vi "Measurement Logic.vi"() -> ()   [LabVIEW 2021, in "audio_adc_acDualChannelMeasurement.lvlib"]
uses:
  audio_adc_acDualChannelMeasurement.lvlib
  Measurement Configuration.ctl
  <vilib>/MeasurementLink/MeasurementLink Measurement Server/Classes/MeasurementContext/MeasurementContext.lvclass
  Measurement Results.ctl
  <vilib>/PDM Acquisition Toolkit/host/Classes/Tasks/PCM Input/Controls/DVR PCM Input Task.ctl
  <vilib>/PDM Acquisition Toolkit/host/Classes/Tasks/PCM Input/PCM Input Task.lvclass
  shared/controls/Sync Commands.ctl
  sub-vis/Protocol Settings Dual Channel.ctl
  <vilib>/DAQmx/create/channels.llb/DAQmx Create Channel (AO-Voltage-Basic).vi
  <vilib>/DAQmx/configure/timing.llb/DAQmx Timing (Sample Clock).vi
  <vilib>/DAQmx/create/channels.llb/DAQmx Create Channel (AO-FuncGen).vi
  <vilib>/PDM Acquisition Toolkit/host/API/Public/Start/Start PCM Input Task.vi
  <vilib>/PDM Acquisition Toolkit/host/API/Public/Read/Read PCM Input Waveform.vi
  <vilib>/PDM Acquisition Toolkit/host/API/Public/Clear/Clear PCM Input Task.vi
  <resource>/objmgr/daqmx.rc
  <vilib>/PDM Acquisition Toolkit/host/API/PDM Acquisition Toolkit.lvlib
panel:
  out "Measurement Results":T1
  out "Measurement Context out":refnum<class "MeasurementContext.lvclass">
  in  "Measurement Context":refnum<class "MeasurementContext.lvclass">
  in  "Measurement Configuration":T2={"Band start"=20.0, "Band stop"=20000.0, "Weighting filter"="", "Amplitude"=1.0, "Frequency"=1000.0, "Full scale range"=2.825, "Analog source resource name"="", "Protocol capture resource name"="", "Data line"=0, "Sample rate"=12288000.0, "Measurement duration"=19200.0, "Channel"="0L", "Frame sync edge for channel 0"=0, "Channel count per frame"=2, "Channel length"=32, "Bit depth"=24, "Channel 0 offset"=1, "Endianness"=0, "Data justification"=0, "Frame length"=64, "Frame sync pulse width"=32, "Bit clock edge sync"=1}
  out "error out":errorcluster
  in  "error in":errorcluster
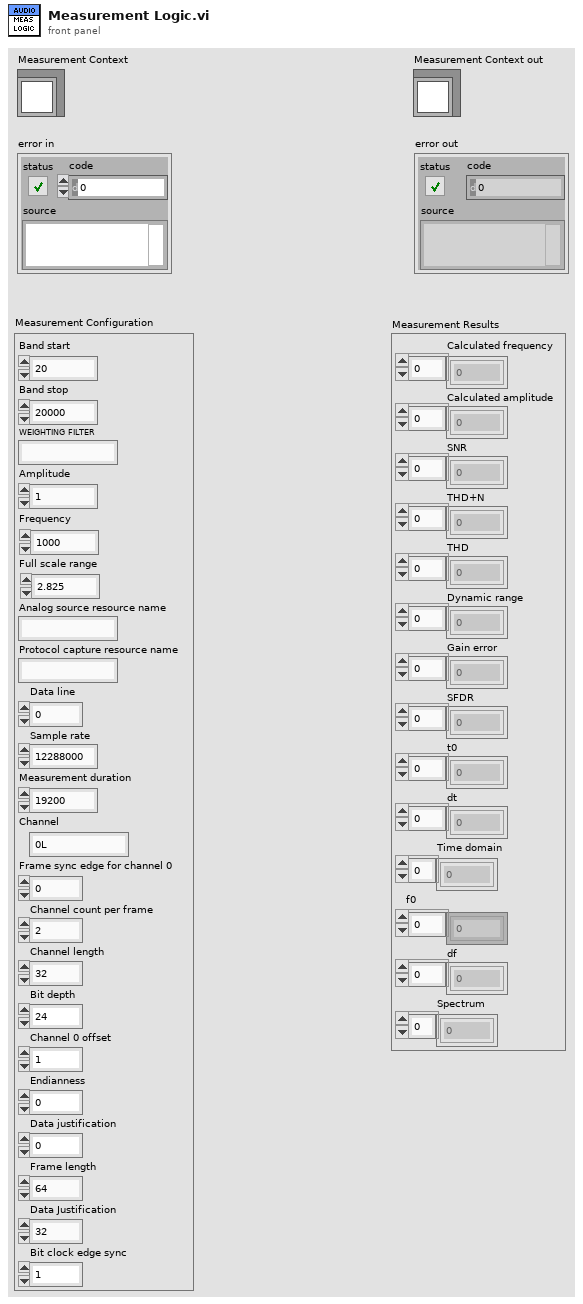
[diagram p1: front panel]
types:
  T1 = typedef "audio_adc_acDualChannelMeasurement.lvlib/Measurement Results.ctl" = cluster{"Calculated frequency":dbl[], "Calculated amplitude":dbl[], "SNR":dbl[], "THD+N":dbl[], "THD":dbl[], "Dynamic range":dbl[], "Gain error":dbl[], "SFDR":dbl[], "t0":dbl[], "dt":dbl[], "Time domain":dbl[], "f0":dbl[], "df":dbl[], "Spectrum":dbl[]}
  T2 = typedef "audio_adc_acDualChannelMeasurement.lvlib/Measurement Configuration.ctl" = cluster{"Band start":dbl, "Band stop":dbl, "Weighting filter":string, "Amplitude":dbl, "Frequency":dbl, "Full scale range":dbl, "Analog source resource name":string, "Protocol capture resource name":string, "Data line":u16, "Sample rate":dbl, "Measurement duration":dbl, "Channel":string, "Frame sync edge for channel 0":u32, "Channel count per frame":u32, "Channel length":u32, "Bit depth":u32, "Channel 0 offset":u32, "Endianness":u32, "Data justification":u32, "Frame length":u32, "Frame sync pulse width":u32, "Bit clock edge sync":u32}
  T3 = typedef "Sync Commands.ctl" = enum16{"NoAction", "GenerationStarted", "AcquisitionCompleted", "GenerationErrored"}
  T4 = typedef "PDM Acquisition Class Library.lvlib/PCM Input Task.lvclass/DVR PCM Input Task.ctl" = refnum<data-value>
  T5 = cluster{"DSG Session":refnum<k21>, "PDM task":T4, "Measurement Results":T1}
  T6 = typedef "audio_adc_acDualChannelMeasurement.lvlib/Protocol Settings Dual Channel.ctl" = cluster{"Protocol capture resource name":string, "Data line":u16, "Channel":string, "Clock rate":u32, "Number of words":i32, "Sensitivity":dbl, "Frame sync edge for channel 0":enum32{"Rising", "Falling"}, "Channel count per frame":u8, "Channel length":u16, "Bit depth":u8, "Channel 0 offset":u16, "Endianness":enum32{"MSB First", "LSB First"}, "Data justification":enum32{"Left Justified", "Right Justified"}, "Frame length":u16, "Frame sync pulse width":u16, "Bit clock edge sync":enum32{"Rising", "Falling"}}
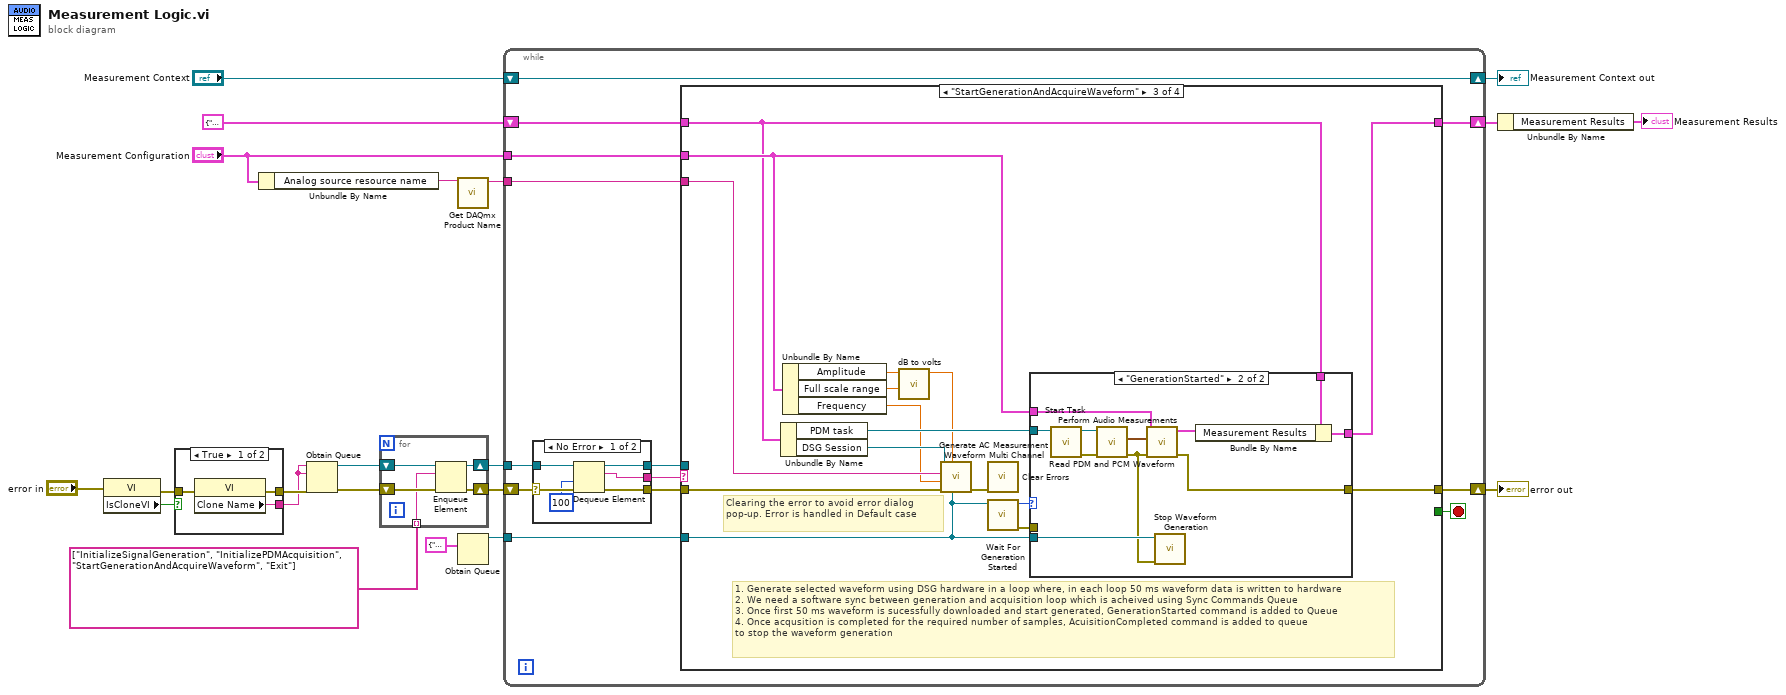
[diagram p0: block diagram]
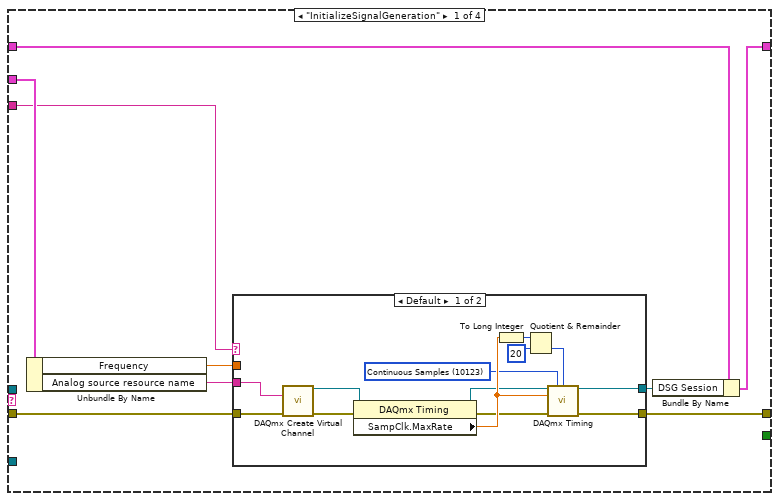
[diagram p2: hidden frame]
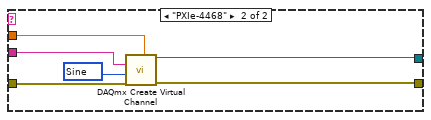
[diagram p3: hidden frame]
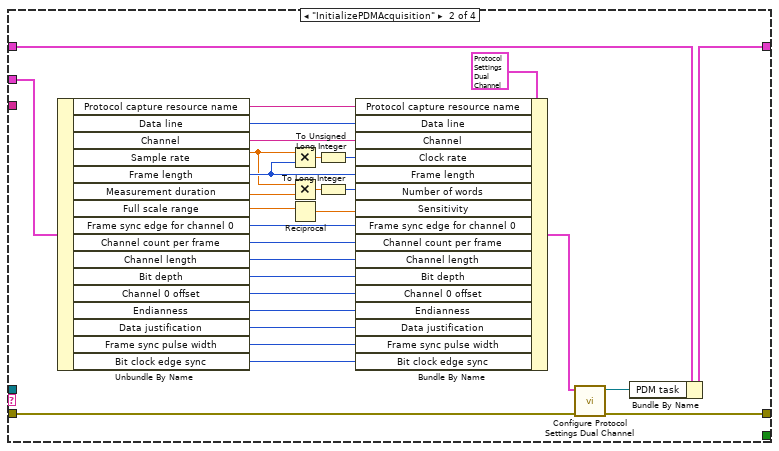
[diagram p4: hidden frame]
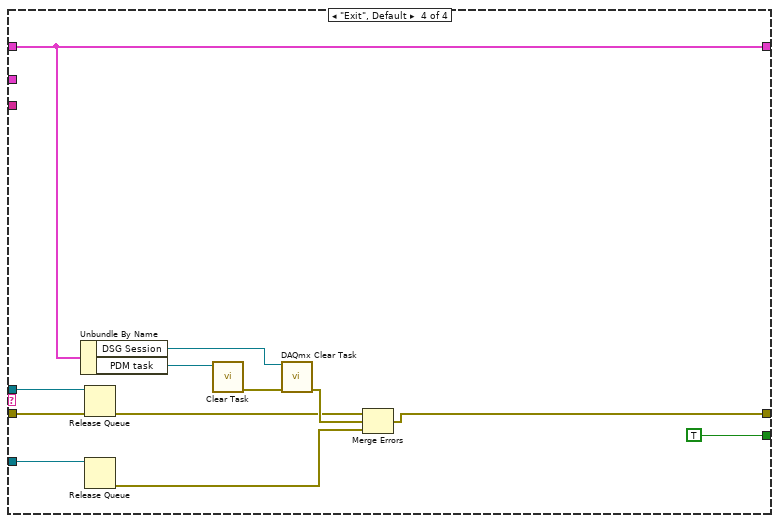
[diagram p6: hidden frame]
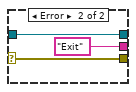
[diagram p7: hidden frame]
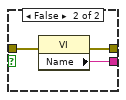
[diagram p8: hidden frame]
diagram:
  n1 = property class="VI"(error in="error in") -> (error out=w19:errorcluster, "IsCloneVI"=w20:bool)  [unwired: 1 in, 1 out]
  n2 = case shown="True" w20 {
    tunnel: [w24 w27] -> w18
    tunnel: [w23 w26] -> w1
    tunnel: w19 -> [w22 w25]
    frame True {
      n3 = property class="VI"(error in=w22) -> (error out=w24:errorcluster, "Clone Name"=w23:string)  [unwired: 1 in, 1 out]
    }
    frame False {
      n4 = property class="VI"(error in=w25) -> (error out=w27:errorcluster, "Name"=w26:string)  [unwired: 1 in, 1 out]
    }
  }
  n5 = Unbundle By Name("Measurement Configuration") -> ("Analog source resource name"=w10:string)
  n6 = Obtain Queue(name (unnamed)=w1, element data type=w1, error in (no error)=w18) -> (queue out=w21:refnum<queue>, error out=w17:errorcluster)  [unwired: 2 in, 1 out]
  n7 = for {
    shift-right: [w30] -> w16
    shift-left: w21 -> [w32]
    shift-right: [w29] -> w15
    shift-left: w17 -> [w31]
    tunnel: string[] ["InitializeSignalGeneration", "InitializePDMAcquisition", "StartGenerationAndAcquireWaveform", "Exit"] ("Step sequence") -> [w28] mode=indexing
    n8 = Enqueue Element(queue=w32, element=w28, error in (no error)=w31) -> (queue out=w30:refnum<queue>, error out=w29:errorcluster)  [unwired: 1 in, 1 out]
  }
  n9 = call "Get DAQmx Product Name.vi"("DAQmx resource name"=w10) -> ("DAQmx product type"=w8:string)  [unwired: 10 in]
  n10 = Obtain Queue(element data type=cluster{"Status":T3, "Error":errorcluster} {"Status"=enum."NoAction", "Error"={"status"=FALSE, "code"=0, "source"=""}}) -> (queue out=w2:refnum<queue>)  [unwired: 4 in, 2 out]
  n11 = while {
    tunnel: w16 -> [w45]
    shift-right: [w42] -> w6
    shift-left: w15 -> [w41]
    shift-right: [w38] -> w11
    shift-left: "Measurement Context" -> [w38]
    tunnel: "Measurement Configuration" -> [w39]
    shift-right: [w36] -> w5
    shift-left: T5 {"DSG Session"="", "PDM task"=refnum, "Measurement Results"={"Calculated frequency"=[], "Calculated amplitude"=[], "SNR"=[], "THD+N"=[], "THD"=[], "Dynamic range"=[], "Gain error"=[], "SFDR"=[], "t0"=[], "dt"=[], "Time domain"=[], "f0"=[], "df"=[], "Spectrum"=[]}} -> [w40]
    tunnel: w8 -> [w35]
    tunnel: w2 -> [w34]
    stop <- w37 stop-if-true
    n12 = case shown="No Error" w41 {
      selector: w41 -> [w147 w151]
      tunnel: w45 -> [w149 w150]
      tunnel: [w148 "Exit" ("t")] -> w44
      tunnel: [w146 w151] -> w43
      tunnel: [w144 w150] -> w33
      frame No Error {
        n13 = Dequeue Element(queue=w149, timeout in ms (-1)=100, error in (no error)=w147) -> (queue out=w144:refnum<queue>, element=w148:string, error out=w146:errorcluster)  [unwired: 1 out]
      }
      frame Error {
      }
    }
    n14 = case shown="\"StartGenerationAndAcquireWaveform\"" w44 {
      tunnel: w43 -> [w53 w97 w117 w133]
      tunnel: [w52 w100 w115 w137] -> w42
      tunnel: w39 -> [w49 w98 w113 _]
      tunnel: w40 -> [w51 w102 w105 w142]
      tunnel: [w50 w101 w104 w142] -> w36
      tunnel: [_ _ _ TRUE] -> w37
      tunnel: w35 -> [w47 _ w114 _]
      tunnel: w34 -> [_ _ w103 w136]
      tunnel: w33 -> [_ _ _ w134]
      frame "InitializeSignalGeneration" {
        # "Generate the sinle tone waveform using an Analog I/O"
        n15 = Unbundle By Name(w49) -> ("Frequency"=w48:dbl, "Analog source resource name"=w54:string)
        n16 = case shown="Default" w47 {
          tunnel: w54 -> [w67 w71]
          tunnel: w53 -> [w66 w73]
          tunnel: [w65 w72] -> w52
          tunnel: [w55 w68] -> w46
          tunnel: w48 -> [_ w69]
          frame Default {
            w56 = 10123 items=["Finite Samples"=10178, "Continuous Samples"=10123, "Hardware Timed Single Point"=12522] ("sample mode")
            n17 = call-poly <vilib>:"DAQmx Create Virtual Channel.vi"("physical channels"=w67, "error in"=w66) -> ("task out"=w64:refnum<k21>, "error out"=w63:errorcluster)  [unwired: 12 in]
            n18 = property class="DAQmx Timing"(reference=w64, error in=w63) -> (reference out=w59:refnum<k21>, error out=w60:errorcluster, "SampClk.MaxRate"=w61:dbl)
            n19 = To Long Integer(number=w61) -> (32bit integer=w57:i32)
            n20 = Quotient & Remainder(x=w57, y=20) -> (floor(x/y)=w62:i32)  [unwired: 1 out]
            n21 = call-poly <vilib>:"DAQmx Timing.vi"("task/channels in"=w59, "sample mode"=w56, "samples per channel"=w62, "rate"=w61, "error in"=w60) -> ("task out"=w55:refnum<k21>, "error out"=w65:errorcluster)  [unwired: 9 in]
          }
          frame "PXIe-4468" {
            w70 = 14751 items=["Sine"=14751, "Triangle"=14752, "Square"=14753, "Sawtooth"=14754] ("type")
            n22 = call-poly <vilib>:"DAQmx Create Virtual Channel.vi"("frequency"=w69, "physical channels"=w71, "type"=w70, "error in"=w73) -> ("task out"=w68:refnum<k21>, "error out"=w72:errorcluster)  [unwired: 10 in]
          }
        }
        n23 = Bundle By Name(cluster=w51, "DSG Session"=w46) -> (w50:T5)
      }
      frame "InitializePDMAcquisition" {
        # "Initialize the PDM acquistion input task to acquire the waveform from the DUT"
        n24 = Unbundle By Name(w98) -> ("Protocol capture resource name"=w94:string, "Data line"=w93:u16, "Channel"=w92:string, "Sample rate"=w78:dbl, "Frame length"=w80:u32, "Measurement duration"=w79:dbl, "Full scale range"=w75:dbl, "Frame sync edge for channel 0"=w83:u32, "Channel count per frame"=w91:u32, "Channel length"=w90:u32, "Bit depth"=w89:u32, "Channel 0 offset"=w88:u32, "Endianness"=w87:u32, "Data justification"=w86:u32, "Frame sync pulse width"=w85:u32, "Bit clock edge sync"=w84:u32)
        n25 = Multiply(x=w78, y=w80) -> (x*y=w82:dbl)
        n26 = Multiply(x=w78, y=w79) -> (x*y=w77:dbl)
        n27 = Reciprocal(x=w75) -> (1/x=w74:dbl)
        n28 = To Unsigned Long Integer(number=w82) -> (unsigned 32bit integer=w81:u32)
        n29 = To Long Integer(number=w77) -> (32bit integer=w76:i32)
        n30 = Bundle By Name(cluster=T6 {"Protocol capture resource name"="", "Data line"=0, "Channel"="", "Clock rate"=12288000, "Number of words"=19200, "Sensitivity"=0.34762, "Frame sync edge for channel 0"=enum."Falling", "Channel count per frame"=2, "Channel length"=32, "Bit depth"=24, "Channel 0 offset"=1, "Endianness"=enum."MSB First", "Data justification"=enum."Left Justified", "Frame length"=64, "Frame sync pulse width"=32, "Bit clock edge sync"=enum."Falling"} ("Protocol settings"), "Protocol capture resource name"=w94, "Data line"=w93, "Channel"=w92, "Clock rate"=w81, "Frame length"=w80, "Number of words"=w76, "Sensitivity"=w74, "Frame sync edge for channel 0"=w83, "Channel count per frame"=w91, "Channel length"=w90, "Bit depth"=w89, "Channel 0 offset"=w88, "Endianness"=w87, "Data justification"=w86, "Frame sync pulse width"=w85, "Bit clock edge sync"=w84) -> (w95:T6)
        n31 = call "Configure Protocol Settings Dual Channel.vi"("error in"=w97, "Protocol settings"=w95) -> ("error out"=w100:errorcluster, "PDM task"=w99:T4)  [unwired: 8 in]
        n32 = Bundle By Name(cluster=w102, "PDM task"=w99) -> (w101:T5)
      }
      frame "StartGenerationAndAcquireWaveform" {
        # "1. Generate selected waveform using DSG hardware in a loop where, in each loop 50 ms waveform data is written to hardware\n2. We need a software sync between generation and acquisition loop which is acheived using Sync Commands Queue\n3. Once first 50 ms waveform is sucessfully downloaded and start generated, GenerationStarted command is added to Queue\n4. Once acqusition is completed for the required number of samples, AcuisitionCompleted command is added to queue\nto stop the waveform generation"
        # "Clearing the error to avoid error dialog pop-up. Error is handled in Default case"
        # "Start the single tone waveform generation and aquire the waveform using PDM toolkit"
        n33 = Unbundle By Name(w105) -> ("PDM task"=w118:T4, "DSG Session"=w116:refnum<k21>)
        n34 = Unbundle By Name(w113) -> ("Amplitude"=w112:dbl, "Full scale range"=w111:dbl, "Frequency"=w109:dbl)
        n35 = call "dB to volts.vi"("Full scale range"=w111, "Voltage(dB)"=w112) -> ("Voltage(volts)"=w110:dbl)  [unwired: 9 in]
        n36 = call "Generate AC Measurement Waveform Multi Channel.vi"("hardware commands sync queue"=w103, "Voltage(volts)"=w110, "error in"=w117, "Frequency"=w109, "DAQmx product name"=w114, "DSG task in"=w116) -> ("error out"=w108:errorcluster)  [unwired: 4 in, 1 out]
        n37 = call <vilib>:"Clear Errors.vi"("error in (no error)"=w108) -> ()  [unwired: 5 in, 2 out]
        n38 = call "Wait For Generation Started.vi"("hardware commands sync queue"=w103) -> ("error out"=w106:errorcluster, "Status"=w107:T3)  [unwired: 9 in]
        n39 = case shown="\"GenerationStarted\"" w107 {
          tunnel: w118 -> [_ w129]
          tunnel: [w120 w121] -> w115
          tunnel: w113 -> [_ w127]
          tunnel: w106 -> [w120 _]
          tunnel: w105 -> [w119 w126]
          tunnel: [w119 w124] -> w104
          tunnel: w103 -> [_ w123]
          frame Default {
          }
          frame "GenerationStarted" {
            n40 = call-poly <vilib>:"Start Task.vi"("PCM input task in"=w129) -> ("error out"=w131:errorcluster, "PCM input task out"=w130:T4)  [unwired: 9 in]
            n41 = call-poly <vilib>:"Read PDM and PCM Waveform.vi"("error in"=w131, "PCM input task In"=w130) -> ("error out"=w122:errorcluster, "PCM waveforms"=w128:waveform(dbl)[])  [unwired: 4 in, 4 out]
            n42 = call "Perform Audio Measurements.vi"("Measurement Configuration"=w127, "I2S waveforms"=w128, "error in"=w122) -> ("Measurement Results"=w125:T1, "error out"=w121:errorcluster)  [unwired: 6 in]
            n43 = call "Stop Waveform Generation.vi"("error in (no error)"=w122, "Hw sync command Q"=w123) -> ()  [unwired: 10 in]
            n44 = Bundle By Name(cluster=w126, "Measurement Results"=w125) -> (w124:T5)
          }
        }
      }
      frame "Exit", Default {
        n45 = Unbundle By Name(w142) -> ("DSG Session"=w141:refnum<k21>, "PDM task"=w140:T4)
        n46 = Release Queue(queue=w134, error in (no error)=w133) -> (error out=w132:errorcluster)  [unwired: 1 in, 2 out]
        n47 = Release Queue(queue=w136) -> (error out=w135:errorcluster)  [unwired: 2 in, 2 out]
        n48 = call-poly <vilib>:"Clear Task.vi"("PCM input task in"=w140) -> ("error out"=w143:errorcluster)  [unwired: 10 in]
        n49 = call <vilib>:"DAQmx Clear Task.vi"("task in"=w141, "error in"=w143) -> ("error out"=w138:errorcluster)  [unwired: 13 in]
        n50 = Merge Errors(w132, w138, w135) -> (w137:errorcluster)
      }
    }
  }
  "error out" <- w6
  "Measurement Context out" <- w11
  n51 = Unbundle By Name(w5) -> ("Measurement Results"=→"Measurement Results":T1)
